vi "duty cycle to wait time.vi"(10 "Frequency [Hz]":dbl=1.0 format="%#_13g", 11 "Duty Cycle [%]":dbl=10.0 format="%#_13g") -> (2 "Off Time [ms]":u32, 3 "On Time [ms]":u32)   [LabVIEW 2025, in "hardware.lvclass"]
uses:
  hardware.lvclass
  hardware.lvclass/hardware.ctl
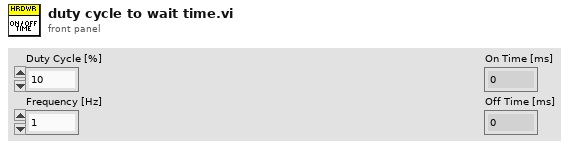
[diagram p1: front panel]
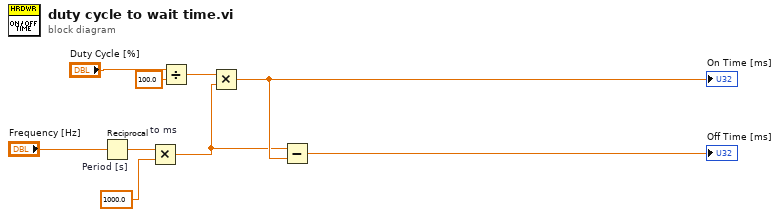
[diagram p0: block diagram]
diagram:
  n1 = Reciprocal "Period [s]"(x="Frequency [Hz]") -> (1/x=w4:dbl)
  n2 = Multiply "to ms"(x=w4, y=1000.0) -> (x*y=w3:dbl)
  n3 = Divide(x="Duty Cycle [%]", y=100.0) -> (x/y=w6:dbl)
  n4 = Multiply(x=w6, y=w3) -> (x*y=w5:dbl)
  "On Time [ms]" <- w5
  n5 = Subtract(x=w3, y=w5) -> (x-y=→"Off Time [ms]":dbl)
